vi "Actor Core.vi"(8 "Error in":errorcluster, 11 "Histogram in":refnum<class "Histogram.lvclass">) -> (0 "error out":errorcluster, 3 "Actor out":refnum<class "Actor.lvclass">)   [LabVIEW 2016, in "Tests.lvlib" / "Histogram.lvclass"]
doc: "This VI helps to view the Pixel distribution of a grayscale image which is nothing but the Histograph."
uses:
  Histogram.lvclass
  C:/Program Files (x86)/National Instruments/LabVIEW 2016/vi.lib/ActorFramework/Actor/Actor.lvclass
  <vilib>/ActorFramework/Actor/Actor.lvclass
  <vilib>/vision/Image Controls.llb/IMAQ Image.ctl
  Histogram Messages/New Image for Histogram Msg/New Image for Histogram Msg.lvclass
  C:/Users/Achu/Desktop/2015/Image Acquisition/Image Acquisition Messages/Image Msg/Image Msg.lvclass
  Controls/Histogram States.ctl
  Histogram.lvclass/Histogram.ctl
  <vilib>/ActorFramework/Actor/Actor.lvclass/Actor.ctl
  <vilib>/ActorFramework/Message Enqueuer/Message Enqueuer.lvclass/Message Enqueuer.ctl
  Controller/Controller Messages/Request Image Msg/Request Image Msg.lvclass/Request Image Msg.ctl
  <vilib>/ActorFramework/Report Error Msg/Report Error Msg.lvclass/Report Error Msg.ctl
  <vilib>/ActorFramework/Message Enqueuer/Init from Existing Queue.vi
  <vilib>/ActorFramework/Message Enqueuer/Enqueue.vi
  Controller/Controller Messages/Request Image Msg/Request Image Msg.lvclass
  C:/Program Files (x86)/National Instruments/LabVIEW 2016/vi.lib/ActorFramework/Message/Message.lvclass
  <vilib>/ActorFramework/Report Error Msg/Report Error Msg.lvclass
  Histogram Messages/Stop Histogram Actor Msg/Stop Histogram Actor Msg.lvclass
  <vilib>/ActorFramework/Stop Msg/Stop Msg.lvclass
  <vilib>/ActorFramework/Message Priority Queue/Priority Enqueue.vi
  Tests.lvclass
  <vilib>/ActorFramework/Message Enqueuer/Message Enqueuer.lvclass
  <vilib>/vision/NI_Vision_Development_Module.lvlib
panel:
  in  "Tests.lvlib:New Image for Histogram Msg.lvclass":refnum<class "New Image for Histogram Msg.lvclass">
  in  "Help Button":bool
  out "New Image from Acquistion Actor":T1
  out "Standard  Deviation":sgl format="%.2f"
  out "Mean Value":sgl format="%.2f"
  in  "View Histograph":bool
  in  "Send Image Request":bool
  out "Histograph":T2(graph)
  out "Image":T1(plugin-control)
  # "Histograph Viewer"
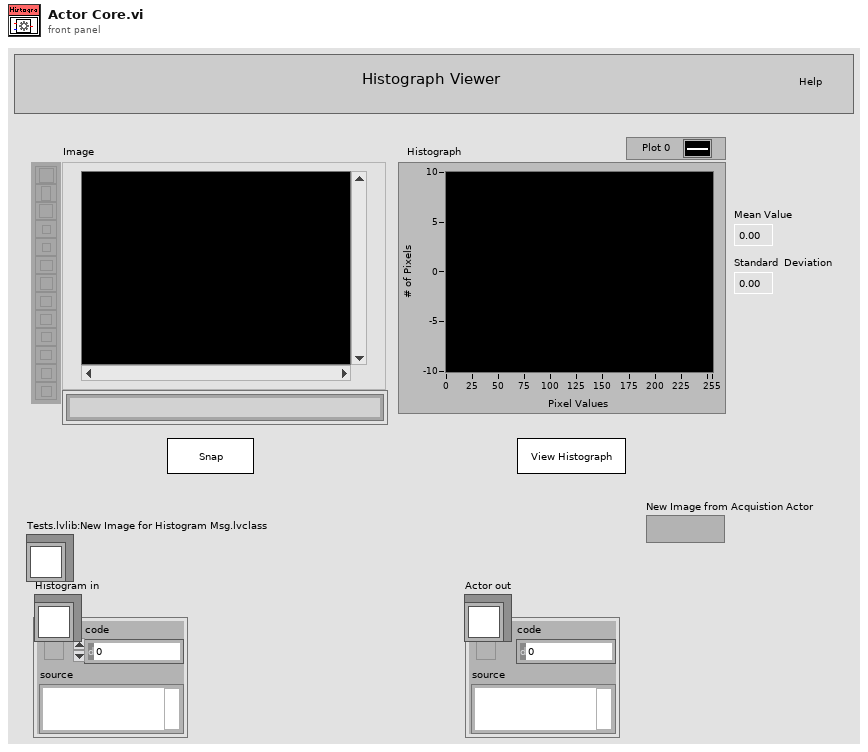
[diagram p1: front panel]
types:
  T1 = typedef "IMAQ Image.ctl" = refnum<image>
  T2 = cluster{"Starting Value":sgl, "Incremental Value":sgl, "Histogram":u32[]}
  T3 = typedef "Histogram States.ctl" = enum16{"Poll UI", "Initialize", "Send Image Request", "New Image", "Histograph", "Error", "Exit"}
  T4 = enum8{"Enabled", "Disabled", "Disabled and Grayed Out"}
  T5 = typedef "Image Type" = u32
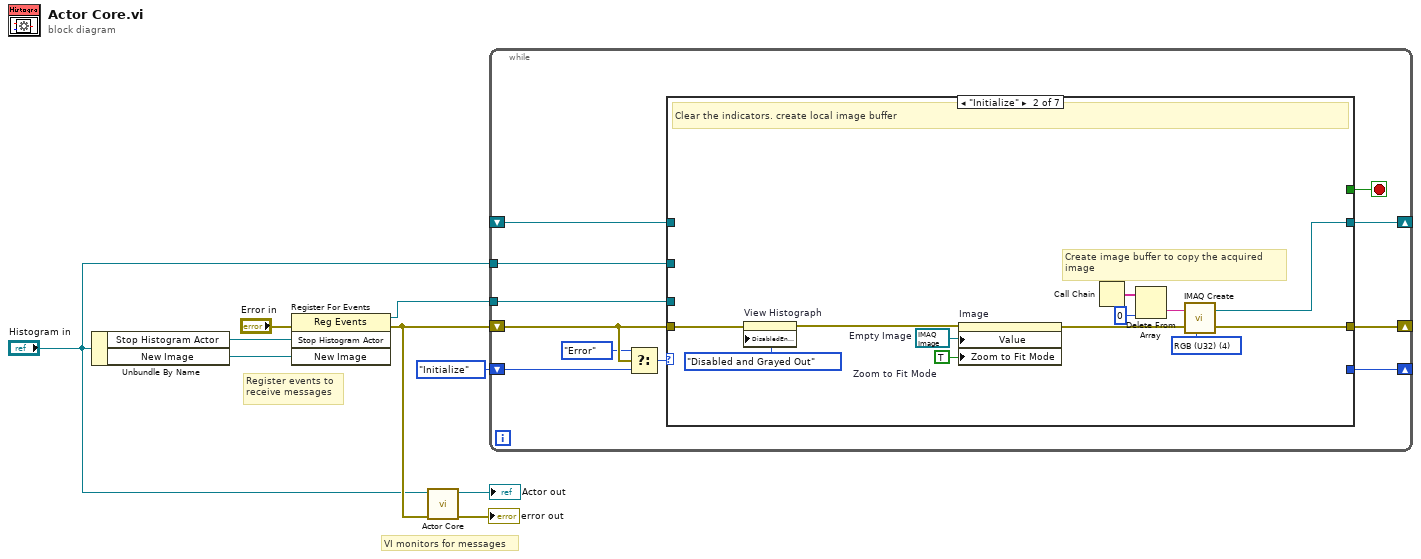
[diagram p0: block diagram]
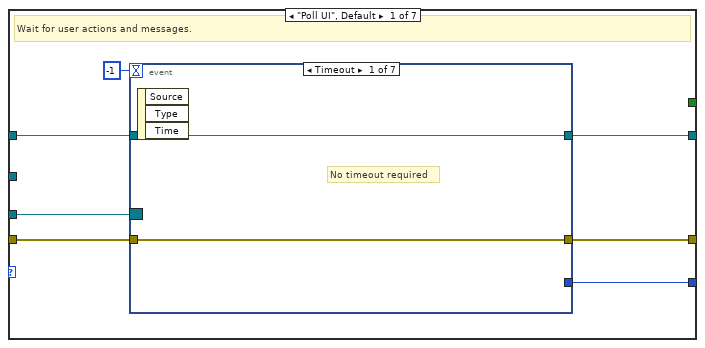
[diagram p2: hidden frame]
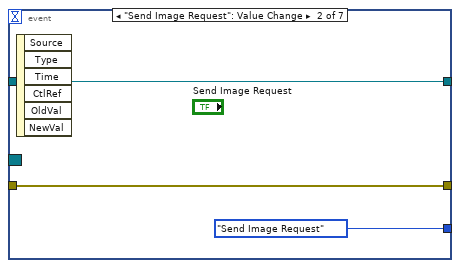
[diagram p3: hidden frame]
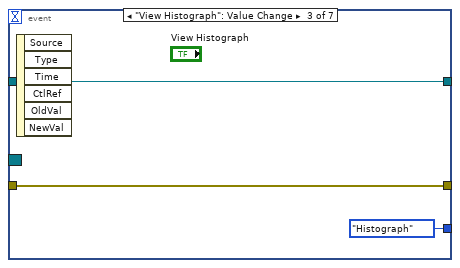
[diagram p4: hidden frame]
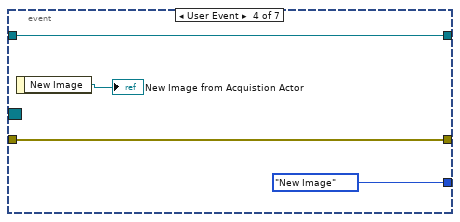
[diagram p5: hidden frame]
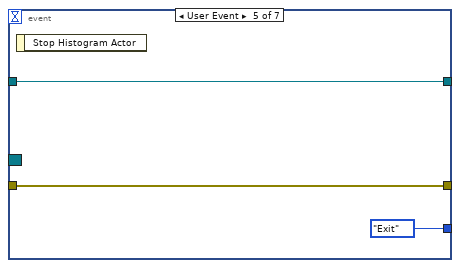
[diagram p6: hidden frame]
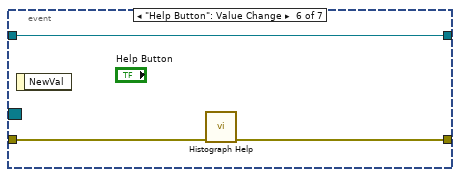
[diagram p7: hidden frame]
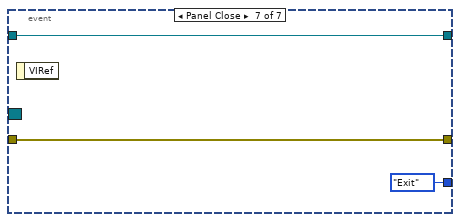
[diagram p8: hidden frame]
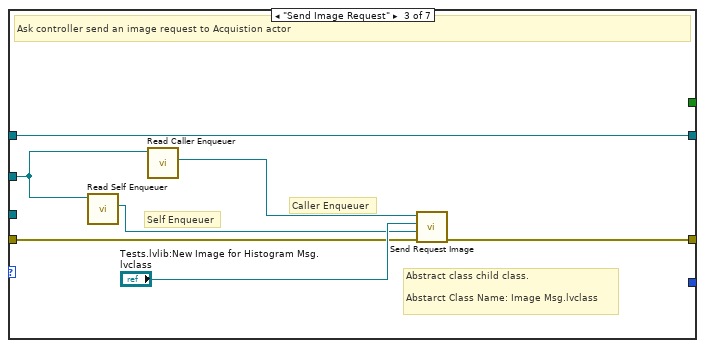
[diagram p9: hidden frame]
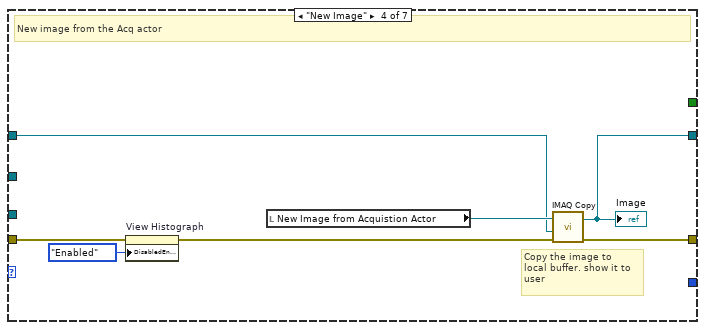
[diagram p10: hidden frame]
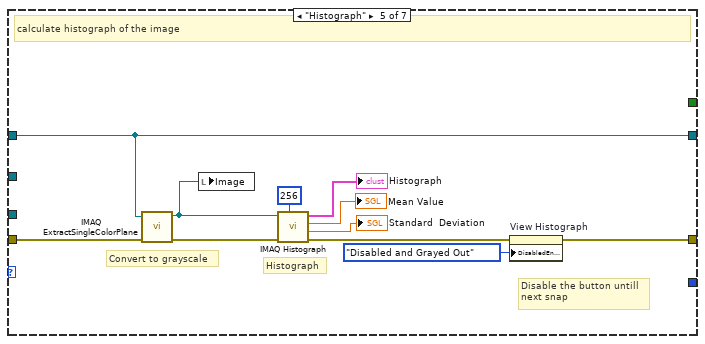
[diagram p11: hidden frame]
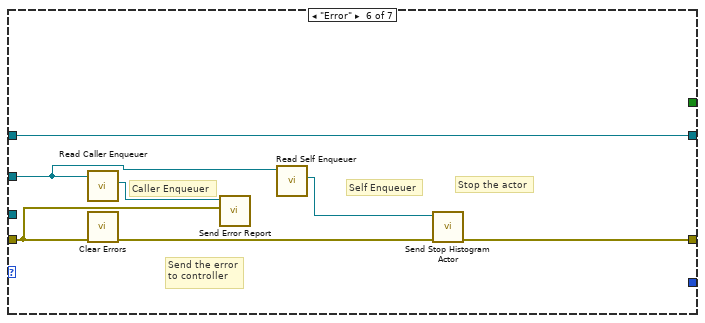
[diagram p12: hidden frame]
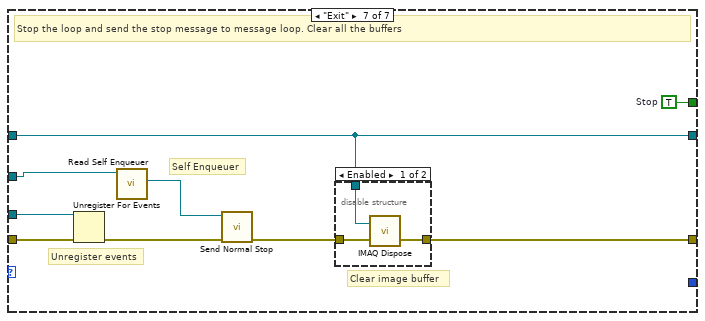
[diagram p13: hidden frame]
diagram:
  # "Register events to \nreceive messages"
  # "VI monitors for messages"
  n1 = Unbundle By Name("Histogram in") -> ("Stop Histogram Actor"=w7:refnum<user-event>, "New Image"=w6:refnum<user-event>)
  n2 = register-events(error in="Error in", w7, w6) -> (reference out=w5:refnum<event-registration>, error out=w3:errorcluster)  [unwired: 1 in]
  n3 = call-parent "Actor Core.vi"("error in"=w3, "Actor in"="Histogram in") -> ("error out"=→"error out":errorcluster, "Actor out"=→"Actor out":refnum<class "Actor.lvclass">)  [unwired: 8 in]
  n4 = while {
    tunnel: w5 -> [w20]
    shift-right: [w19] -> _
    shift-left: w3 -> [w17]
    shift-right: [w18] -> _
    shift-left: Histogram_States."Initialize" -> [w15]
    tunnel: "Histogram in" -> [w13]
    shift-right: [w11] -> _
    shift-left: _ -> [w10]
    stop <- w12 stop-if-true
    n5 = Select(t=Histogram_States."Error", s=w17, f=w15) -> (s? t:f=w14:T3)
    n6 = case shown="\"Initialize\"" w14 {
      tunnel: w20 -> [w27 _ _ _ _ _ w98]
      tunnel: w17 -> [w26 w59 w63 w72 w81 w91 w97]
      tunnel: [w25 w52 w62 w74 w76 w88 w93] -> w19
      tunnel: [w24 _ _ _ _ _ _] -> w18
      tunnel: w13 -> [_ _ w67 _ _ w87 w101]
      tunnel: [_ _ _ _ _ _ w99] -> w12
      tunnel: [w23 w51 w61 w73 w78 w90 w95] -> w11
      tunnel: w10 -> [w22 _ w61 w68 w78 w90 w95]
      frame "Poll UI", Default {
        # "Wait for user actions and messages."
        n7 = event shown="[0] Timeout" {
          selector: w27 -> [_ _ _ _ _ _ _]
          dyn-events: _ -> [_ _ _ _ _ _ _]
          timeout: -1 -> [_ _ _ _ _ _ _]
          tunnel: w26 -> [w29 w32 w35 w39 w42 w44 w48]
          tunnel: [w29 w32 w35 w39 w42 w43 w48] -> w25
          tunnel: [_ Histogram_States."Send Image Request" Histogram_States."Histograph" Histogram_States."New Image" Histogram_States."Exit" _ Histogram_States."Exit"] -> w24
          tunnel: [w28 w30 w34 w37 w40 w45 w46] -> w23
          tunnel: w22 -> [w28 w30 w34 w37 w40 w45 w46]
          event Timeout {
            # "No timeout required"
            n8 = event-data() -> ()  [unwired: 1 in, 3 out]
          }
          event "Send Image Request": Value Change {
            n9 = event-data() -> ()  [unwired: 1 in, 6 out]
          }
          event "View Histograph": Value Change {
            n10 = event-data() -> ()  [unwired: 1 in, 6 out]
          }
          event User Event {
            n11 = event-data() -> ("New Image"=→"New Image from Acquistion Actor":T1)  [unwired: 1 in]
          }
          event User Event {
            n12 = event-data() -> ()  [unwired: 1 in, 1 out]
          }
          event "Help Button": Value Change {
            n13 = event-data() -> ()  [unwired: 1 in, 1 out]
            n14 = call "Histograph Help.vi"("error in (no error)"=w44) -> ("error out"=w43:errorcluster)  [unwired: 10 in]
          }
          event Panel Close {
            n15 = event-data() -> ()  [unwired: 1 in, 1 out]
          }
        }
      }
      frame "Initialize" {
        w49 = TRUE  # Zoom to Fit Mode
        w56 = T5 4 items=["Grayscale (U8)", "Grayscale (I16)", "Grayscale (SGL)", "Complex (CSG)", "RGB (U32)", "HSL (U32)", "RGB (U64)", "Grayscale (U16)"] ("Image Type")
        w57 = T1 refnum  # Empty Image
        # "Create image buffer to copy the acquired \nimage"
        # "Clear the indicators. create local image buffer"
        n16 = property on="View Histograph" class="Bool"(error in=w59, "DisabledEnum"=T4."Disabled and Grayed Out" ("Disabled")) -> (error out=w58:errorcluster)  [unwired: 1 in, 1 out]
        n17 = property on="Image" class="ImageControl"(error in=w58, "Value"=w57, "Zoom to Fit Mode"=w49) -> (error out=w53:errorcluster)  [unwired: 1 in, 1 out]
        n18 = Call Chain() -> (call chain=w54:string[])
        n19 = Delete From Array(array=w54, index=0) -> (deleted portion=w55:string)  [unwired: 1 in, 1 out]
        n20 = call "IMAQ Create"("Image Name"=w55, "Image Type"=w56, "error in (no error)"=w53) -> ("New Image"=w51:T1, "error out"=w52:errorcluster)  [unwired: 2 in]
      }
      frame "Send Image Request" {
        # "Abstract class child class.\n\nAbstarct Class Name: Image Msg.lvclass"
        # "Self Enqueuer"
        # "Caller Enqueuer"
        # "Ask controller send an image request to Acquistion actor"
        n21 = call <vilib>:"Read Self Enqueuer.vi"("Actor"=w67) -> ("Self Enqueuer"=w65:refnum<class "Message Enqueuer.lvclass">)  [unwired: 10 in]
        n22 = call <vilib>:"Read Caller Enqueuer.vi"("Actor"=w67) -> ("Caller Enqueuer"=w64:refnum<class "Message Enqueuer.lvclass">)  [unwired: 10 in]
        n23 = call "Send Request Image.vi"("error in (no error)"=w63, "Enqueuer"=w65, "Image Acquisition.lvlib:Image Msg.lvclass"="Tests.lvlib:New Image for Histogram Msg.lvclass", "Message Enqueuer"=w64) -> ("error out"=w62:errorcluster)  [unwired: 6 in, 1 out]
      }
      frame "New Image" {
        # "Copy the image to \nlocal buffer. show it to\nuser"
        # "New image from the Acq actor"
        n24 = property on="View Histograph" class="Bool"(error in=w72, "DisabledEnum"=T4."Enabled" ("Disabled")) -> (error out=w70:errorcluster)  [unwired: 1 in, 1 out]
        n25 = local read "New Image from Acquistion Actor"() -> (w69:T1)
        n26 = call "IMAQ Copy"("error in (no error)"=w70, "Image Dst"=w68, "Image Src"=w69) -> ("error out"=w74:errorcluster, "Image Dst Out"=w73:T1)  [unwired: 3 in]
        "Image" <- w73
      }
      frame "Histograph" {
        # "Disable the button untill\nnext snap"
        # "Histograph"
        # "Convert to grayscale"
        # "calculate histograph of the image"
        n27 = call "IMAQ ExtractSingleColorPlane"("error in (no error)"=w81, "Image Src"=w78) -> ("error out"=w80:errorcluster, "Image Dst Out"=w79:T1)  [unwired: 8 in]
        n28 = local write "Image"(w79) -> ()
        n29 = call "IMAQ Histograph"("Number of Classes"=256, "error in (no error)"=w80, "Image"=w79) -> ("error out"=w77:errorcluster, "Standard  Deviation"=→"Standard  Deviation":sgl, "Mean Value"=→"Mean Value":sgl, "Histogram Graph"=→"Histograph":T2)  [unwired: 5 in]
        n30 = property on="View Histograph" class="Bool"(error in=w77, "DisabledEnum"=T4."Disabled and Grayed Out" ("Disabled")) -> (error out=w76:errorcluster)  [unwired: 1 in, 1 out]
      }
      frame "Error" {
        # "Caller Enqueuer"
        # "Self Enqueuer"
        # "Send the error\nto controller"
        # "Stop the actor"
        n31 = call <vilib>:"Read Caller Enqueuer.vi"("Actor"=w87) -> ("Caller Enqueuer"=w92:refnum<class "Message Enqueuer.lvclass">)  [unwired: 10 in]
        n32 = call <vilib>:"Clear Errors.vi"("error in (no error)"=w91) -> ("error out"=w89:errorcluster)  [unwired: 5 in, 1 out]
        n33 = call <vilib>:"Send Error Report.vi"("Error From Sender"=w91, "Message Enqueuer"=w92) -> ()  [unwired: 9 in, 1 out]
        n34 = call <vilib>:"Read Self Enqueuer.vi"("Actor"=w87) -> ("Self Enqueuer"=w86:refnum<class "Message Enqueuer.lvclass">)  [unwired: 10 in]
        n35 = call "Send Stop Histogram Actor.vi"("error in (no error)"=w89, "Message Enqueuer"=w86) -> ("error out"=w88:errorcluster)  [unwired: 8 in, 1 out]
      }
      frame "Exit" {
        w99 = TRUE  # Stop
        # "Clear image buffer"
        # "Self Enqueuer"
        # "Unregister events"
        # "Stop the loop and send the stop message to message loop. Clear all the buffers"
        n36 = Unregister For Events(event registration refnum=w98, error in=w97) -> (error out=w96:errorcluster)
        n37 = call <vilib>:"Read Self Enqueuer.vi"("Actor"=w101) -> ("Self Enqueuer"=w100:refnum<class "Message Enqueuer.lvclass">)  [unwired: 10 in]
        n38 = call <vilib>:"Send Normal Stop.vi"("error in (no error)"=w96, "Message Enqueuer"=w100) -> ("error out"=w94:errorcluster)  [unwired: 9 in]
        n39 = disable-structure shown="Enabled" {
          disable-tunnel: w95 -> [w104 _]
          disable-tunnel: w94 -> [w103 w105]
          disable-tunnel: [w102 w105] -> w93
          frame Enabled {
            n40 = call "IMAQ Dispose"("Image"=w104, "error in (no error)"=w103) -> ("error out"=w102:errorcluster)  [unwired: 4 in]
          }
          frame Disabled {
          }
        }
      }
    }
  }
